vi "Host_HoppingScan(YZ_FPGAWithin).vi"() -> ()   [LabVIEW 2014]
uses:
  <vilib>/userdefined/High Color/nirio_resource_hc.ctl
  <vilib>/Native 3D Graph/xcontrol/3DPC_SurfacePlot.xctl
  <vilib>/Instr/_visa.llb/VISA Configure Serial Port (Instr).vi
  <vilib>/FPGAPlugInAG/PCIe-7851R/niLvFpga_Open_PCIe-7851R.vi
  <vilib>/rvi/interface/common/dynamic/niFpgaDynamicAddResources.vi
  <vilib>/Utility/error.llb/Error Cluster From Error Code.vi
  <vilib>/rvi/errors/niLvFpgaAdjustHostInterfaceError.vi
  <vilib>/FPGAPlugInAG/Dynamic/niLvFpga_Close_Dynamic.vi
  <vilib>/rvi/interface/nirviOpenFPGA/nirviOpenFPGA.xnode
  FPGA Bitfiles/XZFPGAWithinHopp_FPGATarget_HoppingStep(Nonl_bBRN9qi7lyY.lvbitx
  <vilib>/rvi/interface/nirviReadWriteControl/nirviReadWriteControl.xnode
  <vilib>/rvi/interface/nirviMethod/nirviMethod.xnode
  <vilib>/rvi/interface/nirviCloseFPGA/nirviCloseFPGA.xnode
  NiFpgaLv.dll
  <vilib>/rvi/interface/Simulation/niFpgaSimulationCallBeginRW.vi
  <vilib>/FPGAPlugInAG/Dynamic/niLvFpga_ReadFifo_Dynamic.vi
  <vilib>/rvi/errors/niLvFpgaMergeErrorWithErrorCode.vi
  <vilib>/FPGAPlugInAG/Dynamic/niLvFpga_StopFifo_Dynamic.vi
panel:
  out "3D Graph":refnum<class "Base Datatype.lvclass">[](xcontrol)
  out "SecElapsed s":dbl
  in  "stop":bool
  out "YBuffer":u32
  out "Waveform Chart":i32(graph)
  out "YGetNum":u32
  in  "Compensation / line":i32
  in  "UseCompensation":bool
  out "YPresPos":i32
  in  "ZOffset index":i32
  out "YPos?":dbl
  in  "PIXDigital":refnum<visa-resource-name>
  out "ERR?":string
  in  "PIYZ":T1
  in  "XInitPos um":dbl format="%#_13g"
  in  "YInitPos um":dbl format="%#_13g"
  in  "YStepMultiplier / 1.5nm":i16
  in  "XStepLen um":dbl format="%#_13g"
  in  "YNum":i16
  in  "XNum":i16
  in  "RelativeWithdraw index":i32
  in  "UpperSleep us":i32
  in  "BottomSleep us":i32
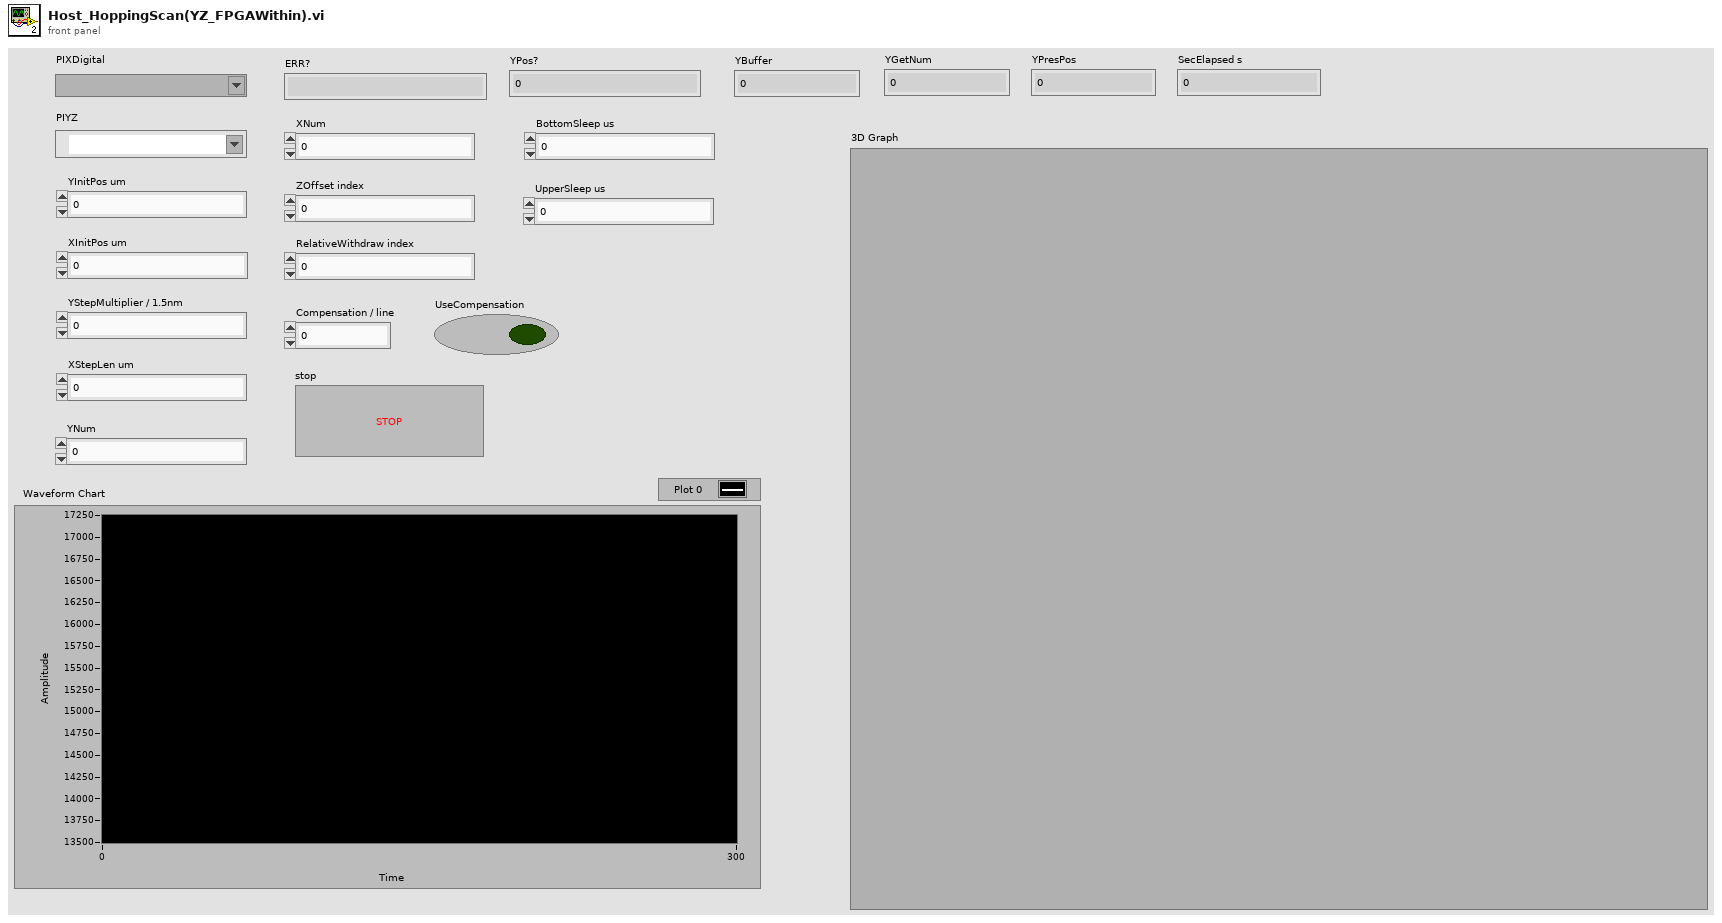
[diagram p1: front panel]
types:
  T1 = typedef "nirio_resource_hc.ctl" = tag
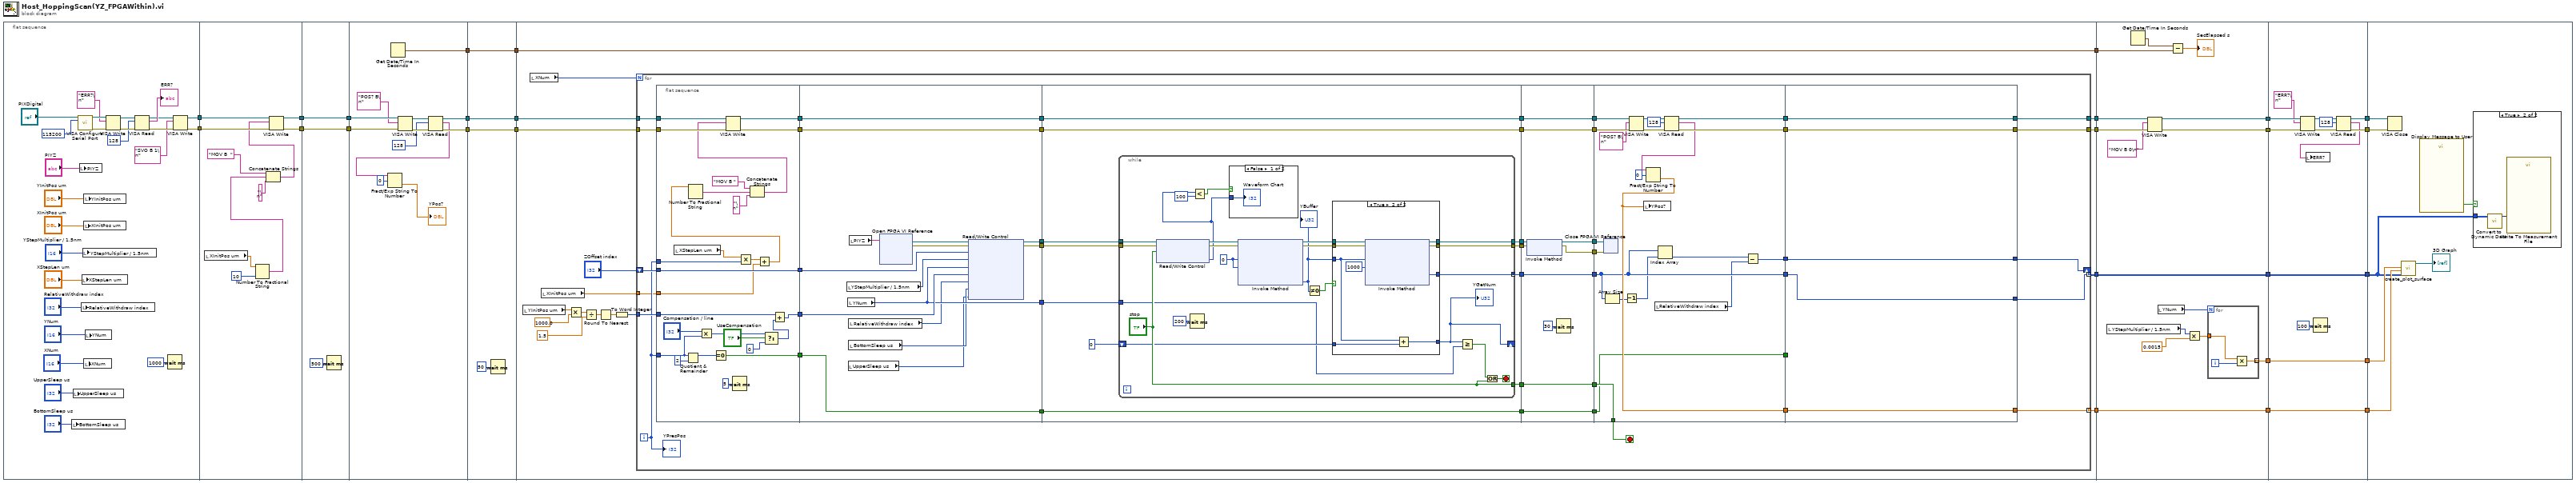
[diagram p0: block diagram]
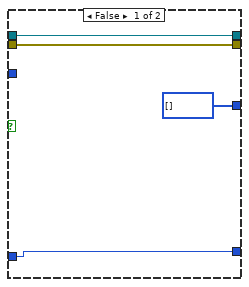
[diagram p3: hidden frame]
diagram:
  n1 = flat-sequence {
    tunnel: [w32] -> w27
    tunnel: [w31] -> w26
    tunnel: w27 -> [w62]
    tunnel: w26 -> [w61]
    tunnel: [w57] -> w25
    tunnel: [w56] -> w24
    tunnel: w25 -> [w64]
    tunnel: w24 -> [w63]
    tunnel: [w64] -> w23
    tunnel: [w63] -> w22
    tunnel: w23 -> [w77]
    tunnel: w22 -> [w76]
    tunnel: [w71] -> w21
    tunnel: [w70] -> w20
    tunnel: [w66] -> w19
    tunnel: w21 -> [w80]
    tunnel: w20 -> [w79]
    tunnel: [w80] -> w18
    tunnel: [w79] -> w17
    tunnel: [w78] -> w16
    tunnel: w19 -> [w78]
    tunnel: w18 -> [w97]
    tunnel: w17 -> [w96]
    tunnel: [w88] -> w15
    tunnel: [w87] -> w14
    tunnel: [w86] -> w13
    tunnel: [w85] -> w12
    tunnel: w16 -> [w82]
    tunnel: [w82] -> w11
    tunnel: w15 -> [w280]
    tunnel: w14 -> [w279]
    tunnel: [w277] -> w10
    tunnel: [w276] -> w9
    tunnel: w13 -> [w269]
    tunnel: w12 -> [w270]
    tunnel: [w271] -> w8
    tunnel: [w270] -> w7
    tunnel: [w269] -> w6
    tunnel: w11 -> [w268]
    tunnel: w10 -> [w296]
    tunnel: w9 -> [w295]
    tunnel: [w290] -> w5
    tunnel: [w289] -> w4
    tunnel: w8 -> [w286]
    tunnel: [w286] -> w3
    tunnel: [w285] -> w2
    tunnel: w7 -> [w285]
    tunnel: [w284] -> w1
    tunnel: w6 -> [w284]
    tunnel: w5 -> [w303]
    tunnel: w4 -> [w302]
    tunnel: w3 -> [w300]
    tunnel: w2 -> [w299]
    tunnel: w1 -> [w297]
    frame #0 {
      n2 = local write "BottomSleep us"("BottomSleep us") -> ()
      n3 = local write "UpperSleep us"("UpperSleep us") -> ()
      n4 = call-poly "VISA Configure Serial Port"("VISA resource name"="PIXDigital", "baud rate (9600)"=u32 115200) -> ("VISA resource name out"=w50:refnum<visa-resource-name>, "error out"=w49:errorcluster)  [unwired: 12 in]
      n5 = local write "PIYZ"("PIYZ") -> ()
      n6 = local write "RelativeWithdraw index"("RelativeWithdraw index") -> ()
      n7 = local write "XStepLen um"("XStepLen um") -> ()
      n8 = local write "YStepMultiplier / 1.5nm"("YStepMultiplier / 1.5nm") -> ()
      n9 = local write "XInitPos um"("XInitPos um") -> ()
      n10 = local write "YInitPos um"("YInitPos um") -> ()
      n11 = local write "XNum"("XNum") -> ()
      n12 = local write "YNum"("YNum") -> ()
      n13 = VISA Write(VISA resource name=w50, write buffer="ERR?\n", error in (no error)=w49) -> (VISA resource name out=w47:refnum<visa-resource-name>, error out=w46:errorcluster)  [unwired: 1 out]
      n14 = VISA Read(VISA resource name=w47, byte count=u32 128, error in (no error)=w46) -> (VISA resource name out=w34:refnum<visa-resource-name>, read buffer=→"ERR?":string, error out=w33:errorcluster)  [unwired: 1 out]
      n15 = Wait (ms)(milliseconds to wait=u32 1000) -> ()  [unwired: 1 out]
      n16 = VISA Write(VISA resource name=w34, write buffer="SVO B 1\n", error in (no error)=w33) -> (VISA resource name out=w32:refnum<visa-resource-name>, error out=w31:errorcluster)  [unwired: 1 out]
    }
    frame #1 {
      n17 = local read "XInitPos um"() -> (w55:dbl)
      n18 = Number To Fractional String(number=w55, precision (6)=i16 10) -> (F-format string=w53:string)  [unwired: 2 in]
      n19 = Concatenate Strings("MOV B  " ("write buffer"), w53, "\n" ("string")) -> (w58:string)
      n20 = VISA Write(VISA resource name=w62, write buffer=w58, error in (no error)=w61) -> (VISA resource name out=w57:refnum<visa-resource-name>, error out=w56:errorcluster)  [unwired: 1 out]
    }
    frame #2 {
      n21 = Wait (ms)(milliseconds to wait=u32 500) -> ()  [unwired: 1 out]
    }
    frame #3 {
      n22 = Get Date/Time In Seconds() -> (seconds since 1Jan1904=w66:timestamp)
      n23 = VISA Write(VISA resource name=w77, write buffer="POS? B\n", error in (no error)=w76) -> (VISA resource name out=w74:refnum<visa-resource-name>, error out=w73:errorcluster)  [unwired: 1 out]
      n24 = VISA Read(VISA resource name=w74, byte count=u32 128, error in (no error)=w73) -> (VISA resource name out=w71:refnum<visa-resource-name>, read buffer=w69:string, error out=w70:errorcluster)  [unwired: 1 out]
      n25 = Fract/Exp String To Number(string=w69, offset=0) -> (number=→"YPos?":dbl)  [unwired: 2 in, 1 out]
    }
    frame #4 {
      n26 = Wait (ms)(milliseconds to wait=u32 50) -> ()  [unwired: 1 out]
    }
    frame #5 {
      n27 = local read "YInitPos um"() -> (w90:dbl)
      n28 = local read "XNum"() -> (w98:i16)
      n29 = local read "XInitPos um"() -> (w83:dbl)
      n30 = Multiply(x=w90, y=1000.0) -> (x*y=w92:dbl)
      n31 = Divide(x=w92, y=1.5) -> (x/y=w94:dbl)
      n32 = Round To Nearest(number=w94) -> (nearest integer value=w95:dbl)
      n33 = To Word Integer(number=w95) -> (16bit integer=w89:i16)
      n34 = for {
        N: w98 -> [_]
        tunnel: w97 -> [w141]
        tunnel: w96 -> [w140]
        tunnel: w89 -> [w134]
        tunnel: [w126] -> w88
        tunnel: [w125] -> w87
        tunnel: [w106] -> w86 mode=indexing
        tunnel: [w117] -> w85 mode=indexing
        shift-right: [w112] -> _
        shift-left: "ZOffset index" -> [w115]
        tunnel: w83 -> [w99]
        i -> [w114]
        stop <- w120 stop-if-true
        n35 = flat-sequence {
          tunnel: w141 -> [w166]
          tunnel: w140 -> [w165]
          tunnel: w114 -> [w167]
          tunnel: [w164] -> w139
          tunnel: [w163] -> w138
          tunnel: [w148] -> w135
          tunnel: w134 -> [w149]
          tunnel: [w157] -> w116
          tunnel: w115 -> [w157]
          tunnel: w114 -> [w146]
          tunnel: [w154] -> w113
          tunnel: w99 -> [w151]
          tunnel: [w179] -> w137
          tunnel: [w178] -> w136
          tunnel: [w174] -> w133
          tunnel: [w173] -> w132
          tunnel: [w175] -> w129
          tunnel: w116 -> [w172]
          tunnel: w135 -> [w176]
          tunnel: w138 -> [w178]
          tunnel: w139 -> [w179]
          tunnel: w113 -> [w171]
          tunnel: [w171] -> w105
          tunnel: w137 -> [w193]
          tunnel: w136 -> [w192]
          tunnel: w133 -> [w185]
          tunnel: w132 -> [w184]
          tunnel: [w193] -> w131
          tunnel: [w192] -> w130
          tunnel: w129 -> [w191]
          tunnel: [w190] -> w128
          tunnel: [w189] -> w127
          tunnel: [w188] -> w122
          tunnel: [w187] -> w118
          tunnel: w105 -> [w186]
          tunnel: [w186] -> w104
          tunnel: w131 -> [w239]
          tunnel: w130 -> [w238]
          tunnel: w128 -> [w234]
          tunnel: w127 -> [w233]
          tunnel: [w239] -> w124
          tunnel: [w238] -> w123
          tunnel: w122 -> [w236]
          tunnel: [w236] -> w121
          tunnel: [w235] -> w119
          tunnel: w118 -> [w235]
          tunnel: w104 -> [w232]
          tunnel: [w232] -> w103
          tunnel: [w231] -> w101
          tunnel: [w230] -> w100
          tunnel: w124 -> [w260]
          tunnel: w123 -> [w259]
          tunnel: w121 -> [w250]
          tunnel: [w250] -> w120
          tunnel: w119 -> [w247]
          tunnel: [w256] -> w111
          tunnel: [w255] -> w110
          tunnel: [w247] -> w109
          tunnel: [w249] -> w108
          tunnel: [w243] -> w107
          tunnel: w103 -> [w242]
          tunnel: [w242] -> w102
          tunnel: w101 -> [w241]
          tunnel: w100 -> [w240]
          tunnel: [w262] -> w112
          tunnel: [w263] -> w117
          tunnel: [w264] -> w125
          tunnel: [w265] -> w126
          tunnel: w111 -> [w265]
          tunnel: w110 -> [w264]
          tunnel: w109 -> [w261]
          tunnel: w108 -> [w263]
          tunnel: w107 -> [w262]
          tunnel: [w261] -> w106
          tunnel: w102 -> [_]
          frame #0 {
            n36 = local read "XStepLen um"() -> (w162:dbl)
            n37 = Quotient & Remainder(x=w146, y=2) -> (x-y*floor(x/y)=w155:i32)  [unwired: 1 out]
            n38 = Multiply(x="Compensation / line", y=w146) -> (x*y=w145:i32)
            n39 = Equal To 0?(x=w155) -> (x = 0?=w154:bool)
            n40 = Wait (ms)(milliseconds to wait=u32 5) -> ()  [unwired: 1 out]
            n41 = Multiply(x=w162, y=w167) -> (x*y=w152:dbl)
            n42 = Add(x=w152, y=w151) -> (x+y=w150:dbl)
            n43 = Number To Fractional String(number=w150) -> (F-format string=w161:string)  [unwired: 3 in]
            n44 = Concatenate Strings("MOV B " ("string"), w161, "\n" ("string")) -> (w158:string)
            n45 = VISA Write(VISA resource name=w166, write buffer=w158, error in (no error)=w165) -> (VISA resource name out=w164:refnum<visa-resource-name>, error out=w163:errorcluster)  [unwired: 1 out]
            n46 = Select(t=w145, s="UseCompensation", f=0) -> (s? t:f=w142:i32)
            n47 = Add(x=w149, y=w142) -> (x+y=w148:i32)
          }
          frame #1 {
            n48 = local read "YStepMultiplier / 1.5nm"() -> (w177:i16)
            n49 = local read "YNum"() -> (w175:i16)
            n50 = local read "UpperSleep us"() -> (w168:i32)
            n51 = local read "RelativeWithdraw index"() -> (w170:i32)
            n52 = local read "BottomSleep us"() -> (w169:i32)
            n53 = local read "PIYZ"() -> (w182:T1)
            n54 = xnode "Open FPGA VI Reference"("resource name"=w182) -> ("FPGA VI Reference Out"=w181:refnum<k20>, "error out"=w180:errorcluster)  [unwired: 1 in]
            n55 = xnode "Read/Write Control"("FPGA VI Reference In"=w181, "error in"=w180, "ZOffset"=w172, "YStepIndex"=w177, "YNum"=w175, "YOffset"=w176, "RelativeWithdraw"=w170, "bottomsleep us"=w169, "uppersleep us"=w168) -> ("FPGA VI Reference Out"=w174:refnum<k20>, "error out"=w173:errorcluster)
          }
          frame #2 {
            n56 = while {
              tunnel: w185 -> [w208]
              tunnel: w184 -> [w207]
              tunnel: w191 -> [w195]
              tunnel: [w211] -> w190
              tunnel: [w210] -> w189
              tunnel: ["stop"] -> w188
              tunnel: [w204] -> w187 mode=concatenating
              shift-right: [w194] -> _
              shift-left: 0 -> [w197]
              stop <- w209 stop-if-true
              w214 = u32 0 ("Number of Elements")
              n57 = xnode "Read/Write Control"("FPGA VI Reference In"=w208, "error in"=w207, "stop"="stop") -> ("FPGA VI Reference Out"=w206:refnum<k20>, "error out"=w205:errorcluster, "Waveform Chart"=w200:i32)
              n58 = Wait (ms)(milliseconds to wait=u32 200) -> ()  [unwired: 1 out]
              n59 = Less?(x=w200, y=100) -> (x < y?=w201:bool)
              n60 = case shown="False" w201 {
                tunnel: w200 -> [w216 _]
                frame False {
                  "Waveform Chart" <- w216
                }
                frame True {
                }
              }
              n61 = xnode "Invoke Method"("FPGA VI Reference In"=w206, "error in"=w205, "Number of Elements"=w214, "Timeout (ms)"=w214) -> ("FPGA VI Reference Out"=w213:refnum<k20>, "error out"=w212:errorcluster, "Elements Remaining"=w198:u32)  [unwired: 1 out]
              "YBuffer" <- w198
              n62 = Not Equal To 0?(x=w198) -> (x != 0?=w199:bool)
              n63 = case shown="True" w199 {
                tunnel: w213 -> [w220 w229]
                tunnel: w212 -> [w219 w228]
                tunnel: [w220 w226] -> w211
                tunnel: [w219 w225] -> w210
                tunnel: [i16[] [] ("Data") w224] -> w204
                tunnel: w198 -> [_ w222]
                tunnel: w197 -> [w217 w223]
                tunnel: [w217 w221] -> w194
                frame False {
                }
                frame True {
                  n64 = xnode "Invoke Method"("FPGA VI Reference In"=w229, "error in"=w228, "Number of Elements"=w222, "Timeout (ms)"=1000) -> ("FPGA VI Reference Out"=w226:refnum<k20>, "error out"=w225:errorcluster, "Data"=w224:i16[])  [unwired: 1 out]
                  n65 = Add(x=w222, y=w223) -> (x+y=w221:u32)
                }
              }
              "YGetNum" <- w194
              n66 = Greater Or Equal?(x=w194, y=w195) -> (x >= y?=w196:bool)
              n67 = Or(x=w196, y="stop") -> (x .or. y?=w209:bool)
            }
          }
          frame #3 {
            n68 = xnode "Invoke Method"("FPGA VI Reference In"=w234, "error in"=w233) -> ("FPGA VI Reference Out"=w231:refnum<k20>, "error out"=w230:errorcluster)
            n69 = Wait (ms)(milliseconds to wait=u32 30) -> ()  [unwired: 1 out]
          }
          frame #4 {
            n70 = xnode "Close FPGA VI Reference"("FPGA VI Reference In"=w241, "error in"=w240) -> ()  [unwired: 1 out]
            n71 = Array Size(array=w247) -> (size(s)=w248:i32)
            n72 = Decrement(x=w248) -> (x-1=w246:i32)
            n73 = VISA Write(VISA resource name=w260, write buffer="POS? B\n", error in (no error)=w259) -> (VISA resource name out=w258:refnum<visa-resource-name>, error out=w257:errorcluster)  [unwired: 1 out]
            n74 = local read "RelativeWithdraw index"() -> (w244:i32)
            n75 = Index Array(array=w247, index=w246) -> (element=w245:i16)
            n76 = VISA Read(VISA resource name=w258, byte count=u32 128, error in (no error)=w257) -> (VISA resource name out=w256:refnum<visa-resource-name>, read buffer=w252:string, error out=w255:errorcluster)  [unwired: 1 out]
            n77 = Fract/Exp String To Number(string=w252, offset=0) -> (number=w249:dbl)  [unwired: 2 in, 1 out]
            n78 = local write "YPos?"(w249) -> ()
            n79 = Subtract(x=w245, y=w244) -> (x-y=w243:i32)
          }
          frame #5 {
          }
        }
        "YPresPos" <- w114
      }
    }
    frame #6 {
      n80 = local read "YStepMultiplier / 1.5nm"() -> (w274:i16)
      n81 = Get Date/Time In Seconds() -> (seconds since 1Jan1904=w267:timestamp)
      n82 = VISA Write(VISA resource name=w280, write buffer="MOV B 0\n", error in (no error)=w279) -> (VISA resource name out=w277:refnum<visa-resource-name>, error out=w276:errorcluster)  [unwired: 1 out]
      n83 = local read "YNum"() -> (w275:i16)
      n84 = Subtract(x=w267, y=w268) -> (x-y=→"SecElapsed s":dbl)
      n85 = Multiply(x=w274, y=0.0015) -> (x*y=w272:dbl)
      n86 = for {
        N: w275 -> [_]
        tunnel: w272 -> [w283]
        tunnel: [w281] -> w271 mode=indexing
        i -> [w282]
        n87 = Multiply(x=w283, y=w282) -> (x*y=w281:dbl)
      }
    }
    frame #7 {
      n88 = VISA Write(VISA resource name=w296, write buffer="ERR?\n", error in (no error)=w295) -> (VISA resource name out=w293:refnum<visa-resource-name>, error out=w292:errorcluster)  [unwired: 1 out]
      n89 = Wait (ms)(milliseconds to wait=u32 100) -> ()  [unwired: 1 out]
      n90 = VISA Read(VISA resource name=w293, byte count=u32 128, error in (no error)=w292) -> (VISA resource name out=w290:refnum<visa-resource-name>, read buffer=w288:string, error out=w289:errorcluster)  [unwired: 1 out]
      n91 = local write "ERR?"(w288) -> ()
    }
    frame #8 {
      n92 = VISA Close(VISA resource name=w303, error in (no error)=w302) -> ()  [unwired: 1 out]
      n93 = call <vilib>:"create_plot_surface.vi"("z matrix"=w297, "y vector"=w299, "x vector"=w300) -> ("plots out"=→"3D Graph":refnum<class "Base Datatype.lvclass">[])  [unwired: 2 in, 6 out]
      n94 = call "Display Message to User"() -> ("OK"=w298:bool)  [unwired: 10 in, 1 out]
      n95 = case shown="True" w298 {
        tunnel: w297 -> [_ w305]
        frame False {
        }
        frame True {
          n96 = call "Convert to Dynamic Data"("2D Array"=w305) -> ("Dynamic Data Type"=w304:dynamicdata)  [unwired: 3 in]
          n97 = call "Write To Measurement File"("Signals"=w304) -> ()  [unwired: 16 in, 3 out]
        }
      }
    }
  }
